vi "FTW-Endpoint-TCP-Connection-Set.vi"(8 "error in (no error)":errorcluster, 10 "Connection":refnum<k5>, 11 "FTW-Endpoint-TCP in":refnum<class "FTW-Endpoint-TCP.lvclass">) -> (0 "error out":errorcluster, 3 "FTW-Endpoint-TCP out":refnum<class "FTW-Endpoint-TCP.lvclass">)   [LabVIEW 2015, in "FTW-Endpoint-TCP.lvclass"]
uses:
  FTW-Endpoint-TCP.lvclass
  FTW-Endpoint-TCP.lvclass/FTW-Endpoint-TCP.ctl
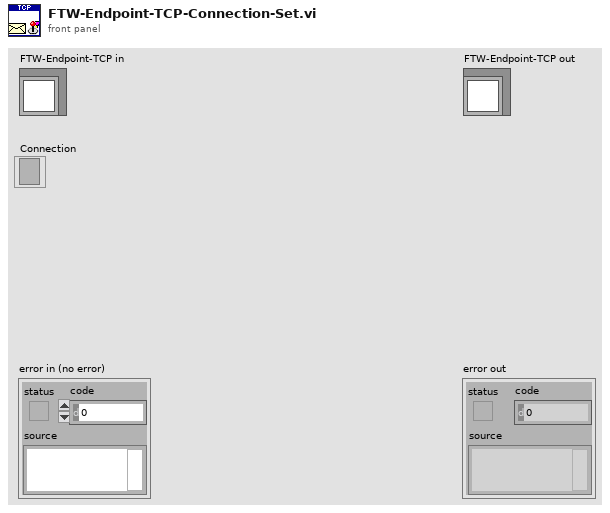
[diagram p1: front panel]
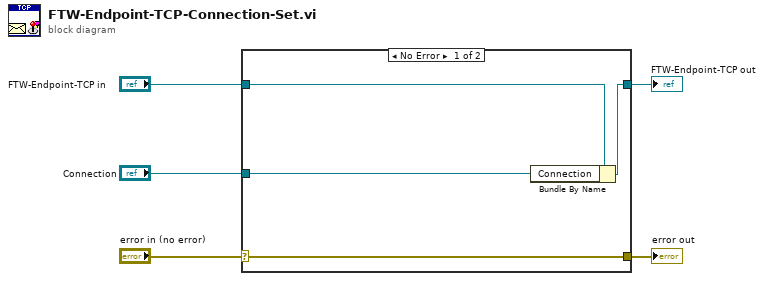
[diagram p0: block diagram]
diagram:
  n1 = case shown="No Error" "error in (no error)" {
    selector: "error in (no error)" -> [w9 w10]
    tunnel: [w9 w10] -> w4
    tunnel: [w7 w11] -> w2
    tunnel: "FTW-Endpoint-TCP in" -> [w8 w11]
    tunnel: "Connection" -> [w6 _]
    frame No Error {
      n2 = Bundle By Name(cluster=w8, "Connection"=w6) -> (w7:refnum<class "FTW-Endpoint-TCP.lvclass">)
    }
    frame Error {
    }
  }
  "error out" <- w4
  "FTW-Endpoint-TCP out" <- w2
